vi "TopLevel.vi"() -> ()   [LabVIEW 2023]
uses:
  Test-Programs/LabVIEW Data/Common VIs/Logging/TDMSFileProperties.ctl
  <vilib>/drjdpowell/Messenging/Core Messengers/EventMessenger/EventMessenger.lvclass
  C:/Program Files (x86)/National Instruments/LabVIEW 2023/vi.lib/drjdpowell/Messenging/Core Messengers/Send/Send.lvclass
  <vilib>/drjdpowell/Messenging/Useful Actors/Metronome/Metronome.lvclass
  <vilib>/Utility/config.llb/Config Data RefNum.ctl
  <vilib>/drjdpowell/Messenging/Parallel Process/Actor type 2/Actor type2.lvclass
  <vilib>/drjdpowell/Messenging/Core Messages/Message/MSG.lvclass
  Test-Programs/LabVIEW Data/Common VIs/LoggingActor/DataLogger/DataLogger.lvclass
  C:/Program Files (x86)/National Instruments/LabVIEW 2023/vi.lib/drjdpowell/Messenging/Parallel Process/Actor type 2/Actor type2.lvclass
  Test-Programs/LabVIEW Data/HardwareActors/LabJack/LabJack.lvclass
  <vilib>/drjdpowell/Messenging/Observer/Message Translation/LabelPrefix Folder/LabelPrefix.lvclass/LabelPrefix.ctl
  <vilib>/drjdpowell/Messenging/Observer/ObserverSet/ObserverSet.lvclass/ObserverSet.ctl
  <vilib>/drjdpowell/Messenging/Observer/Observer (Parent)/Observer.lvclass/Observer.ctl
  <vilib>/drjdpowell/Messenging/Core Messages/Message/MSG.lvclass/MSG.ctl
  <vilib>/drjdpowell/Messenging/Core Messages/VarMessage/VariantMSG.lvclass/VariantMSG.ctl
  <vilib>/drjdpowell/Messenging/Core Messages/ErrorMessage/ErrorMSG.lvclass/ErrorMSG.ctl
  <vilib>/drjdpowell/Messenging/ObserverRegister/ObserverRegistry.lvclass/ObserverRegistry.ctl
  232e0ddc-f0a7-475d-9058-5032f8458813.vi
  4898256e-b016-494f-9508-2ceef4e6911c.vi
  fbe48fe1-a9cb-4763-93ba-57ead91cbc6a.vi
  <vilib>/drjdpowell/Messenging/Observer/ObserverSet/Prefix Messages.vi
  da9fa938-703e-4c08-9a98-6a32d2093df5.vi
  9b4254ec-8474-4d97-9ca8-57f430c7d8e7.vi
  0a5995e6-4927-490a-bb37-60573358c305.vi
  110a24bf-4286-4484-b55a-b16bf2ec8831.vi
  1f5a9617-5d79-4e61-ab12-c2058fb64140.vi
  cfb725ca-ad06-4a59-ac7e-8d4b7f4c84e1.vi
  9016b64b-a8fb-4694-8e11-e9e188559255.vi
  86903c63-ab96-464e-805c-7ef89f07dfc2.vi
  d424b141-51df-465e-96e3-0435ae11a4e9.vi
  6f407243-e5cf-4ee0-b394-424fafddb9ed.vi
  <vilib>/drjdpowell/Messenging/Core Messages/Message/Read Message Label (faster).vi
  <vilib>/drjdpowell/Messenging/Observer/Message Translation/LabelPrefix Folder/Prefix.vi
  <vilib>/drjdpowell/Messenging/Observer/ObserverSet/Add Translator.vi
  da9fa938-703e-4c08-9a98-6a32d2093df5.vi/afc9f7b6-782e-46b2-95da-8e576e84c933.vi
  9b4254ec-8474-4d97-9ca8-57f430c7d8e7.vi/afc9f7b6-782e-46b2-95da-8e576e84c933.vi
  0a5995e6-4927-490a-bb37-60573358c305.vi/afc9f7b6-782e-46b2-95da-8e576e84c933.vi
  110a24bf-4286-4484-b55a-b16bf2ec8831.vi/afc9f7b6-782e-46b2-95da-8e576e84c933.vi
  1f5a9617-5d79-4e61-ab12-c2058fb64140.vi/afc9f7b6-782e-46b2-95da-8e576e84c933.vi
  cfb725ca-ad06-4a59-ac7e-8d4b7f4c84e1.vi/afc9f7b6-782e-46b2-95da-8e576e84c933.vi
  9016b64b-a8fb-4694-8e11-e9e188559255.vi/afc9f7b6-782e-46b2-95da-8e576e84c933.vi
  86903c63-ab96-464e-805c-7ef89f07dfc2.vi/afc9f7b6-782e-46b2-95da-8e576e84c933.vi
  d424b141-51df-465e-96e3-0435ae11a4e9.vi/afc9f7b6-782e-46b2-95da-8e576e84c933.vi
  6f407243-e5cf-4ee0-b394-424fafddb9ed.vi/afc9f7b6-782e-46b2-95da-8e576e84c933.vi
  <vilib>/drjdpowell/Messenging/Core Messages/Message/Get Label (internal).vi
  <vilib>/drjdpowell/Messenging/Observer/ObserverSet/Write Array of Observers.vi
  <vilib>/drjdpowell/Messenging/Observer/Observer (Parent)/Make Observer.vi
  <vilib>/drjdpowell/Messenging/Core Messages/VarMessage/Write VariantMSG.vi
  <vilib>/drjdpowell/Messenging/Core Messages/Message/Overwrite Reply Address.vi
  <vilib>/drjdpowell/Messenging/Core Messages/Message/Write (no data).vi
  <vilib>/drjdpowell/Messenging/Core Messages/ErrorMessage/Write ErrorMessage.vi
  <vilib>/drjdpowell/Messenging/Core Messages/Message/Label Message.vi
  <vilib>/drjdpowell/Messenging/Observer/Message Translation/LabelPrefix Folder/LabelPrefix.lvclass
  C:/Program Files (x86)/National Instruments/LabVIEW 2023/vi.lib/drjdpowell/Messenging/Observer/Message Translation/Translator/Translator.lvclass
  <vilib>/drjdpowell/Messenging/Observer/ObserverSet/ObserverSet.lvclass
  C:/Program Files (x86)/National Instruments/LabVIEW 2023/vi.lib/drjdpowell/Messenging/Observer/Observer (Parent)/Observer.lvclass
  <vilib>/drjdpowell/Messenging/Observer/Observer (Parent)/Observer.lvclass
  <vilib>/drjdpowell/Messenging/Core Messages/VarMessage/VariantMSG.lvclass
  C:/Program Files (x86)/National Instruments/LabVIEW 2023/vi.lib/drjdpowell/Messenging/Core Messages/Message/MSG.lvclass
  <vilib>/drjdpowell/Messenging/Core Messages/ErrorMessage/ErrorMSG.lvclass
  <vilib>/Utility/config.llb/Read Key (String).vi
  <vilib>/drjdpowell/Messenging/ObserverRegister/Send RegisterForAll.vi
  <vilib>/drjdpowell/Messenging/Observer/Message Translation/Translator/Translator.lvclass
  <vilib>/drjdpowell/Messenging/Core Messengers/Send/Send.lvclass
  <vilib>/drjdpowell/Messenging/ObserverRegister/Commands/ParentCommand/ObserverRegistryCommand.lvclass
  <vilib>/drjdpowell/Messenging/ObserverRegister/ObsReg.lvlib
  <vilib>/drjdpowell/Messenging/Actor Templates Support/Actor Template Support.lvlib
  <vilib>/drjdpowell/Messenging/ObserverRegister/ObserverRegistry.lvclass
  <vilib>/drjdpowell/Messenging/Core Messages/MSG Library/SendMSG.lvlib
  <vilib>/drjdpowell/Messenging/Dialog Boxes/Display Message to User/Async Display Message to User.lvclass
  <vilib>/Utility/config.llb/NI_LVConfig.lvlib
  C:/Program Files (x86)/National Instruments/LabVIEW 2023/vi.lib/drjdpowell/Messenging/Core Messengers/Messenger (Parent)/Messenger.lvclass
  C:/Program Files (x86)/National Instruments/LabVIEW 2023/vi.lib/drjdpowell/Messenging/Core Messengers/EventMessenger/EventMessenger.lvclass
  <vilib>/drjdpowell/Messenging/Observer/Observer (Parent)/Observer.lvlib
  C:/Program Files (x86)/National Instruments/LabVIEW 2023/vi.lib/drjdpowell/Messenging/Parallel Process/Actor/Actor.lvclass
panel:
  in  "Clear Graphs":bool
  in  "Tab Control":enum32{"LabJack"}(tab)
  in  "Pressure Regulator":dbl(slide) caption="PSI" scale=0.0..450.0
  in  "Connect LabJack":bool
  in  "Load":bool
  in  "Default All Current Values":bool
  in  "Reset Elapsed Time":bool
  out "Elapsed Time":dbl format="%<%H:%M:%S>t"
  out "Test In Progress":bool
  in  "End Test":bool
  in  "Start Test":bool
  in  "Test Properties":T1
  in  "Stop":bool
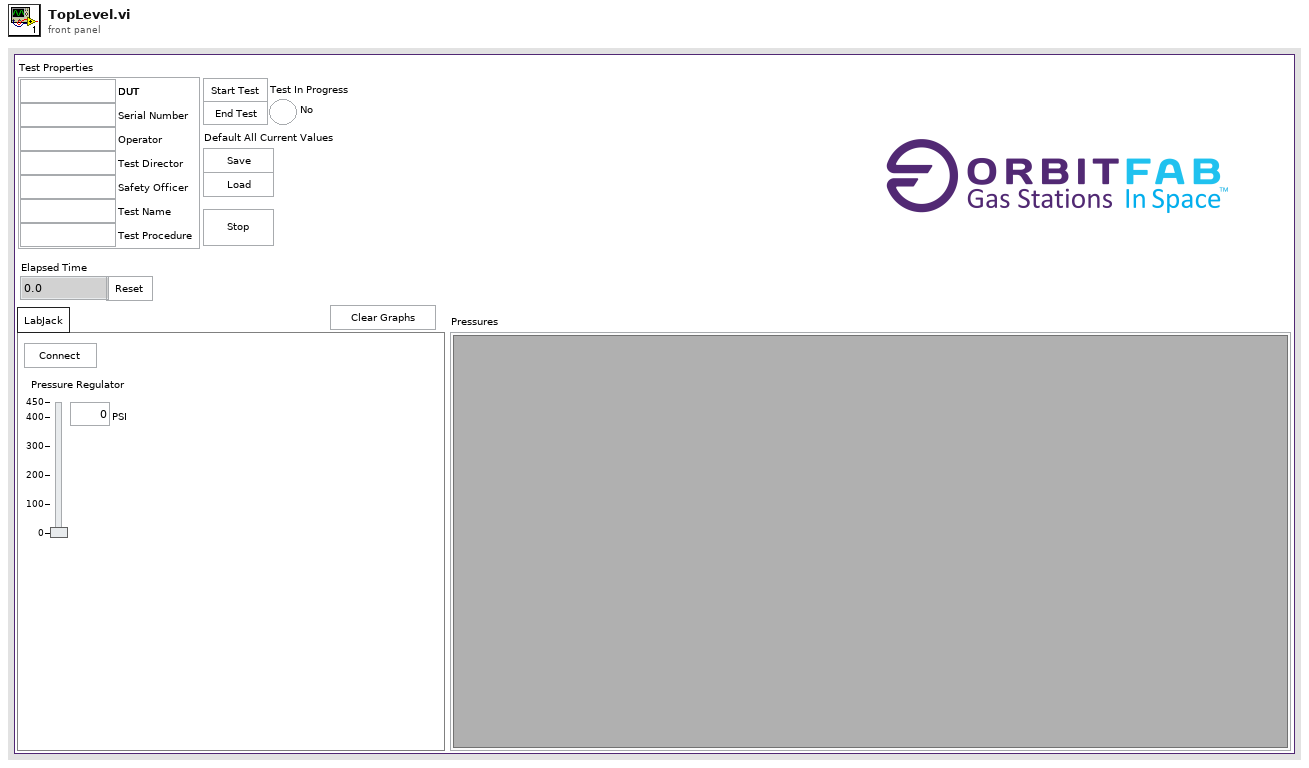
[diagram p1: front panel]
types:
  T1 = typedef "TDMSFileProperties.ctl" = cluster{"DUT":string, "Serial Number":string, "Operator":string, "Test Director":string, "Safety Officer":string, "Test Station":string, "Test Name":string, "Test Procedure":string}
  T2 = typedef "NI_LVConfig.lvlib/Config Data RefNum.ctl" = refnum<k1>
  T3 = cluster{"TopLevelMessenger":refnum<class "EventMessenger.lvclass">, "Test Status":cluster{"Test Metronome":refnum<class "Metronome.lvclass">, "Test Status":string, "Step Time":timestamp}, "App Control":cluster{"Front Panel Config refnum":T2, "This VI":refnum<vi>, "FP Metronome":refnum<class "Metronome.lvclass">, "WFM Data":waveform(dbl)[], "PT Data":dbl[]}, "DataLogger":cluster{"Actor":refnum<class "Actor type2.lvclass">, "Record Data":bool, "Data Packet":cluster{"Group Name":string, "Channel Names":string[], "Data":dbl[]}}, "EmailNotifier":cluster{"Actor":refnum<class "Actor type2.lvclass">, "Send":bool, "Last Sent":timestamp}, "LabJack":cluster{"Actor":refnum<class "Actor type2.lvclass">, "Metronome":refnum<class "Metronome.lvclass">, "Handle":u32, "Connected":bool, "t0":timestamp, "dt":dbl, "PT Data":dbl[][], "Target PSI":dbl, "PT Names":string[], "TDAC#":string}}
  T4 = cluster{"\"Message Received\" Event Reg":refnum<event-registration>}
  T5 = cluster{"Multipliers":dbl[], "Offsets":dbl[], "Names":string[]}
  T6 = cluster{"PT +Channels":string[], "PT -Channels":i32[], "PT Multipliers":dbl[], "PT Offsets":dbl[]}
  T7 = cluster{"Group Name":string, "Channel Names":string[], "Data":dbl[]}
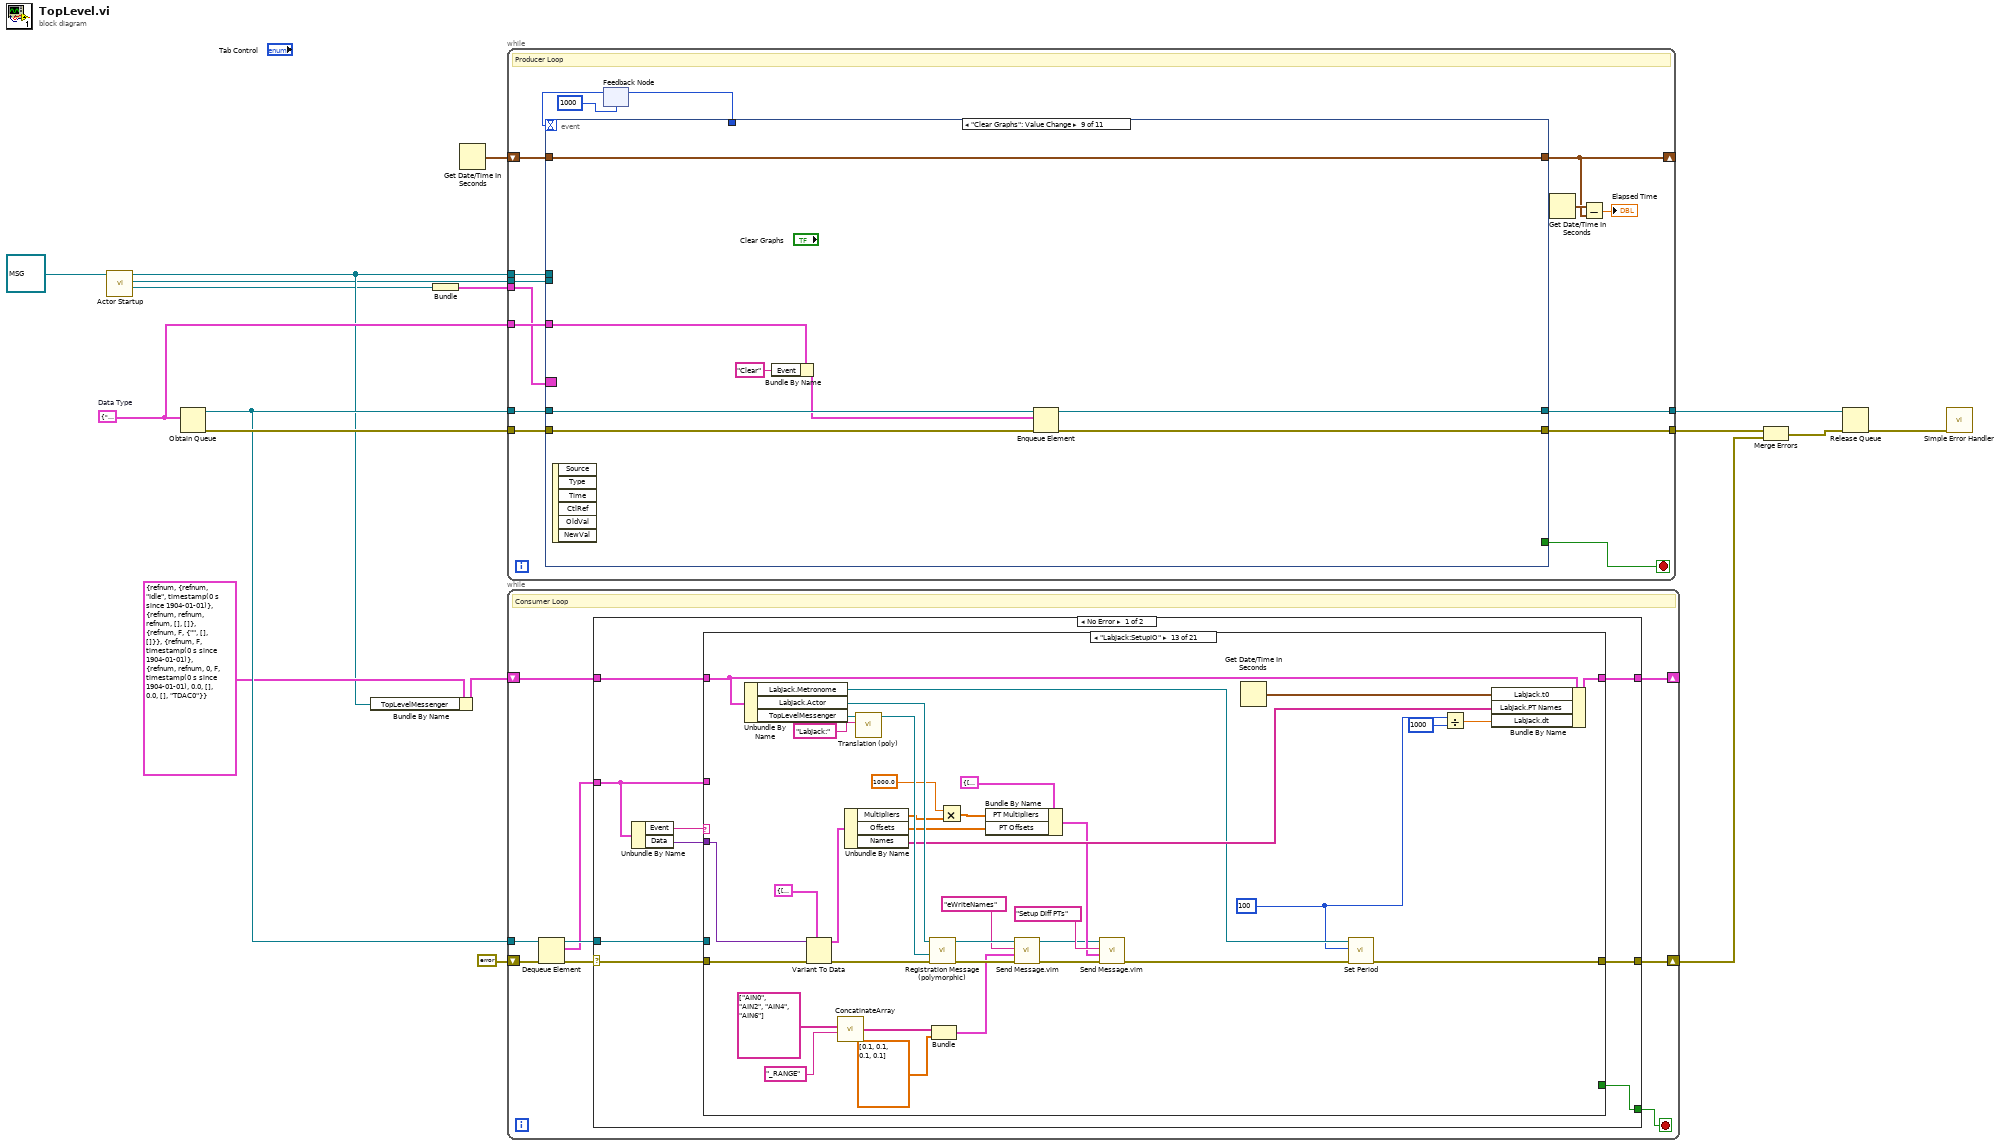
[diagram p0: block diagram]
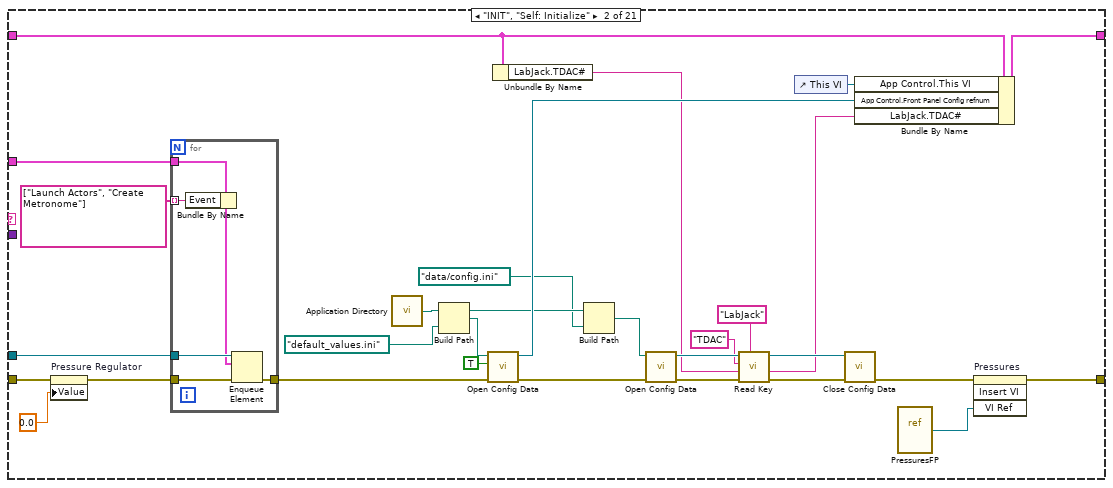
[diagram p3: hidden frame]
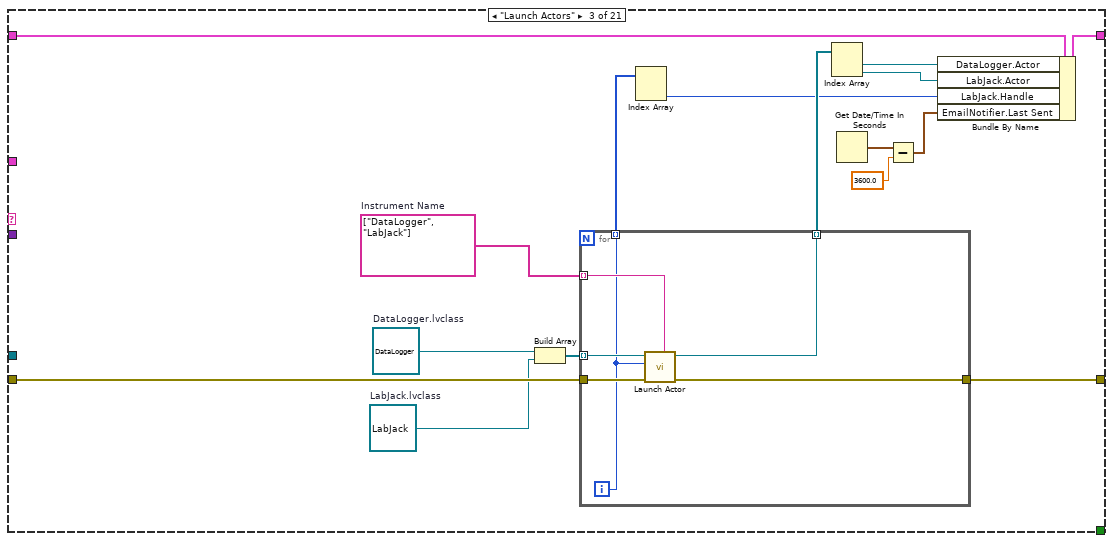
[diagram p4: hidden frame]
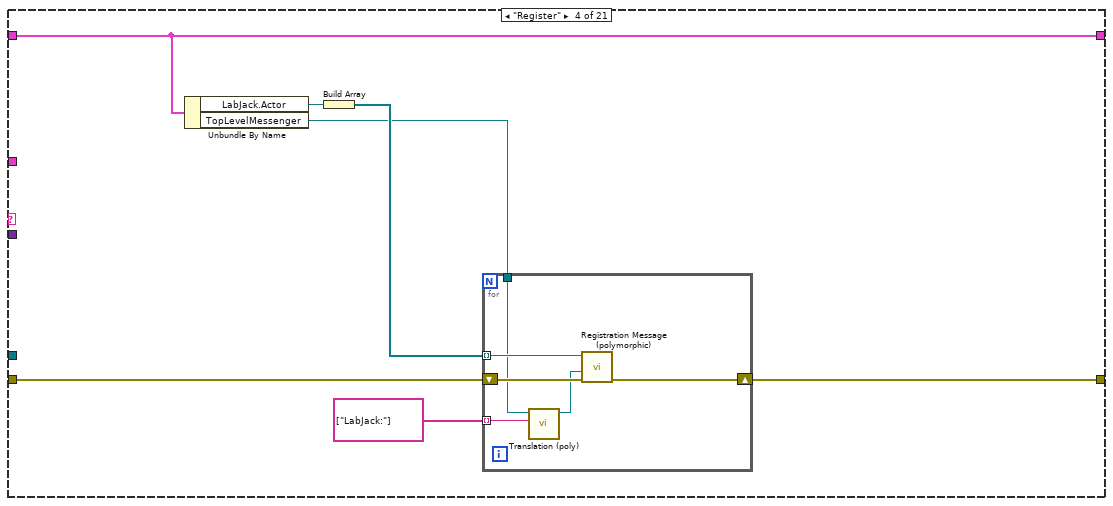
[diagram p5: hidden frame]
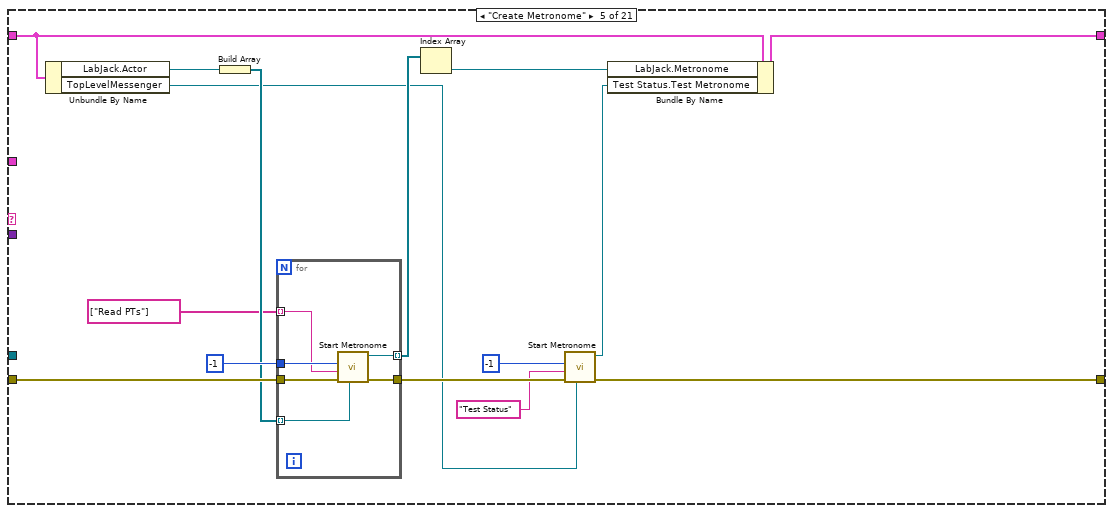
[diagram p6: hidden frame]
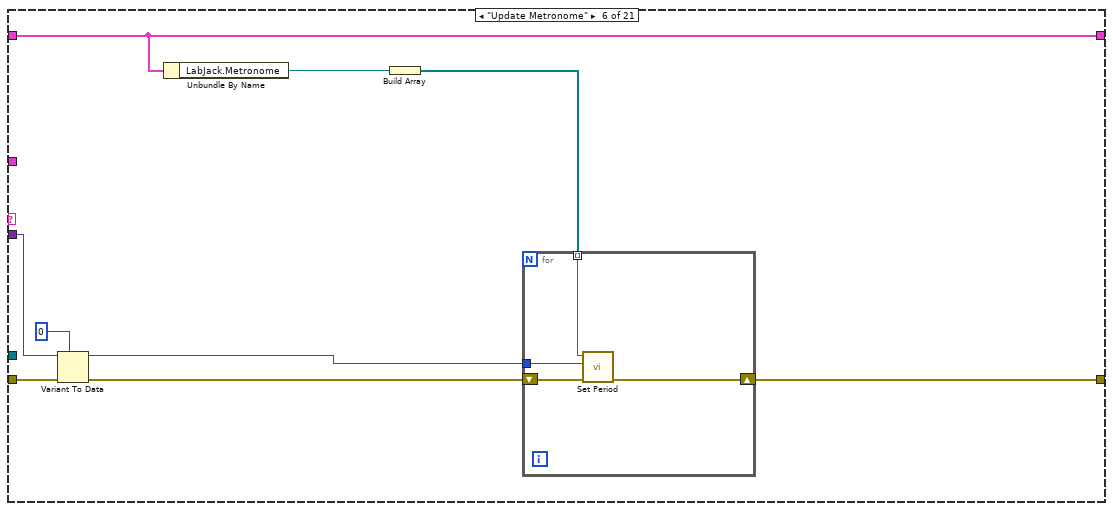
[diagram p7: hidden frame]
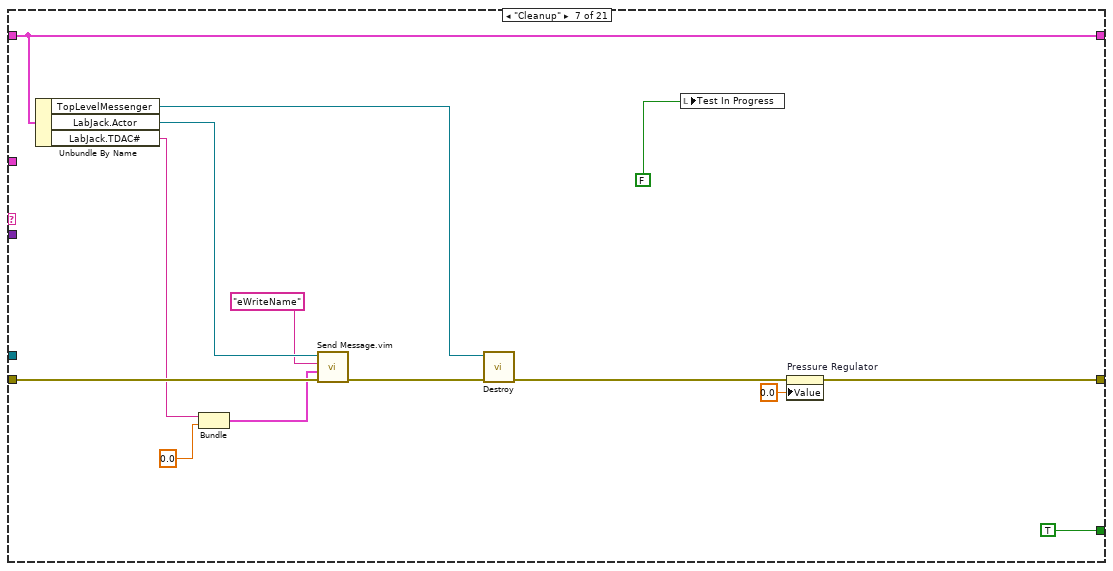
[diagram p8: hidden frame]
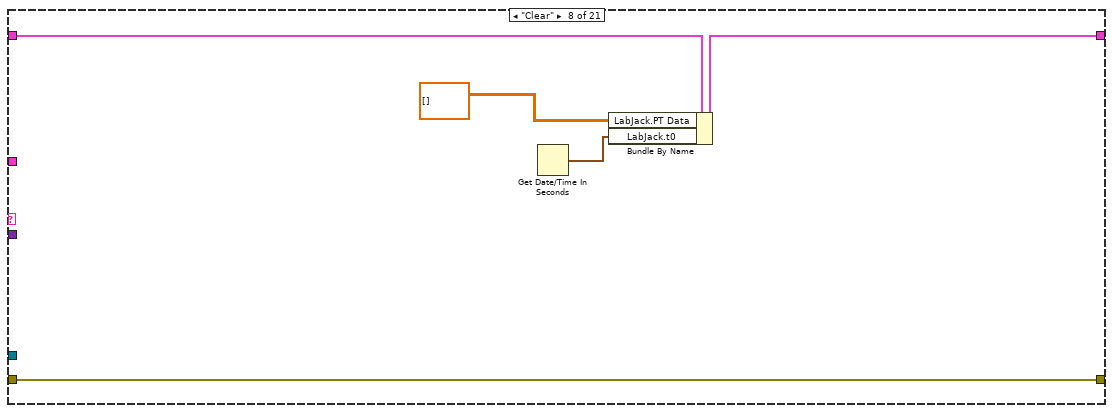
[diagram p9: hidden frame]
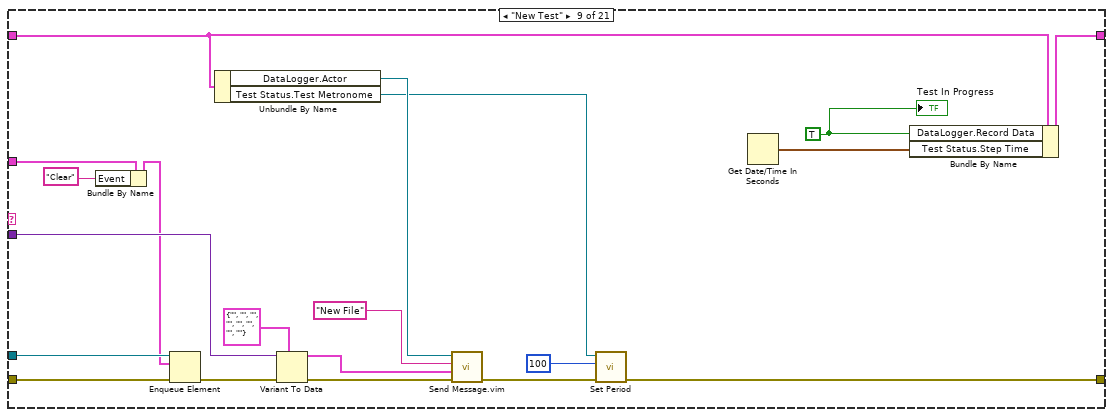
[diagram p10: hidden frame]
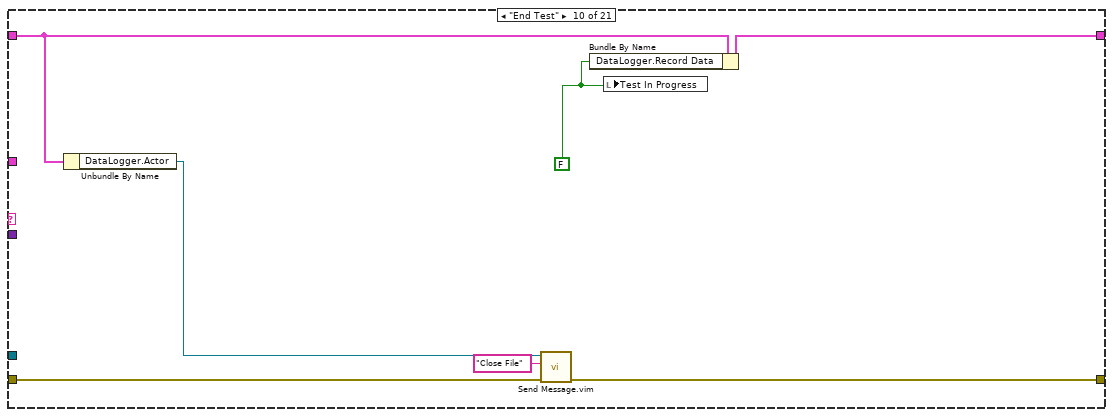
[diagram p11: hidden frame]
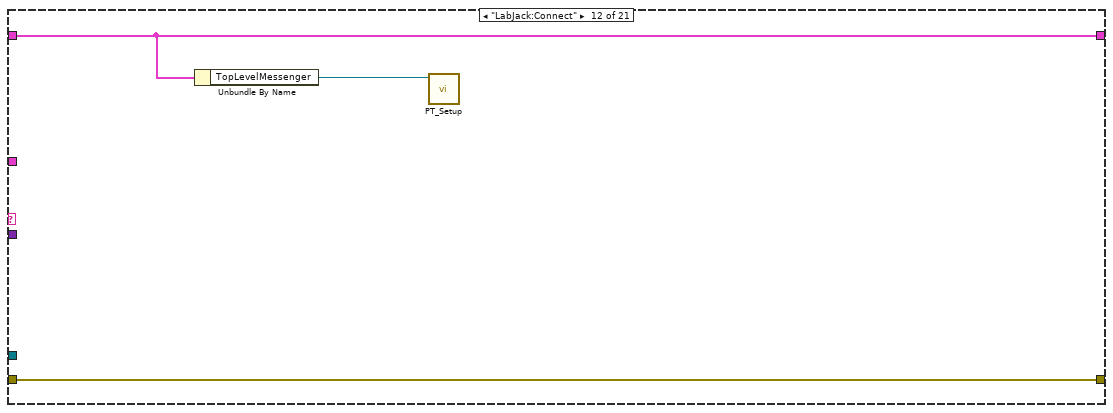
[diagram p13: hidden frame]
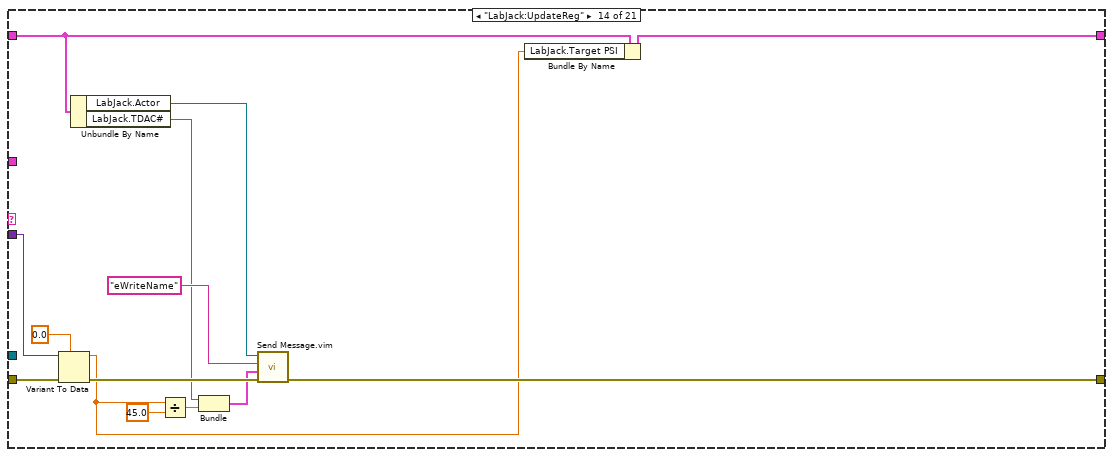
[diagram p14: hidden frame]
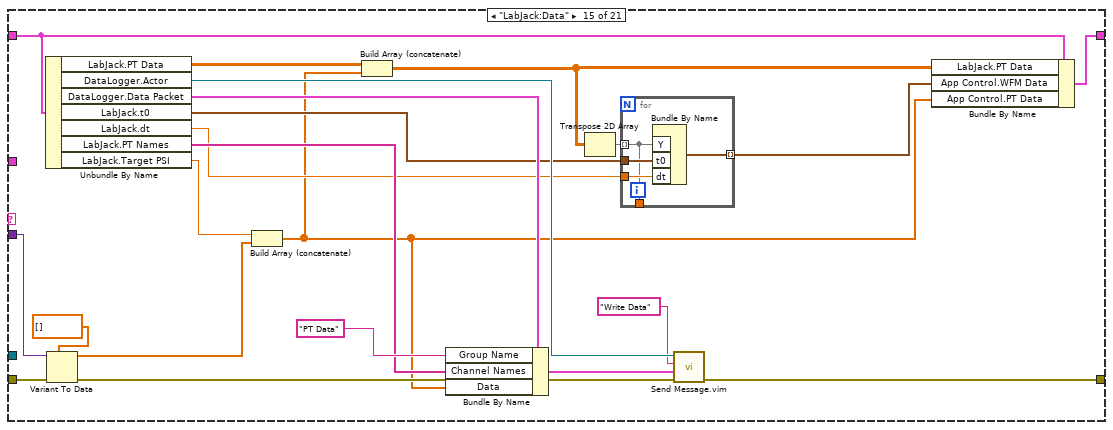
[diagram p15: hidden frame]
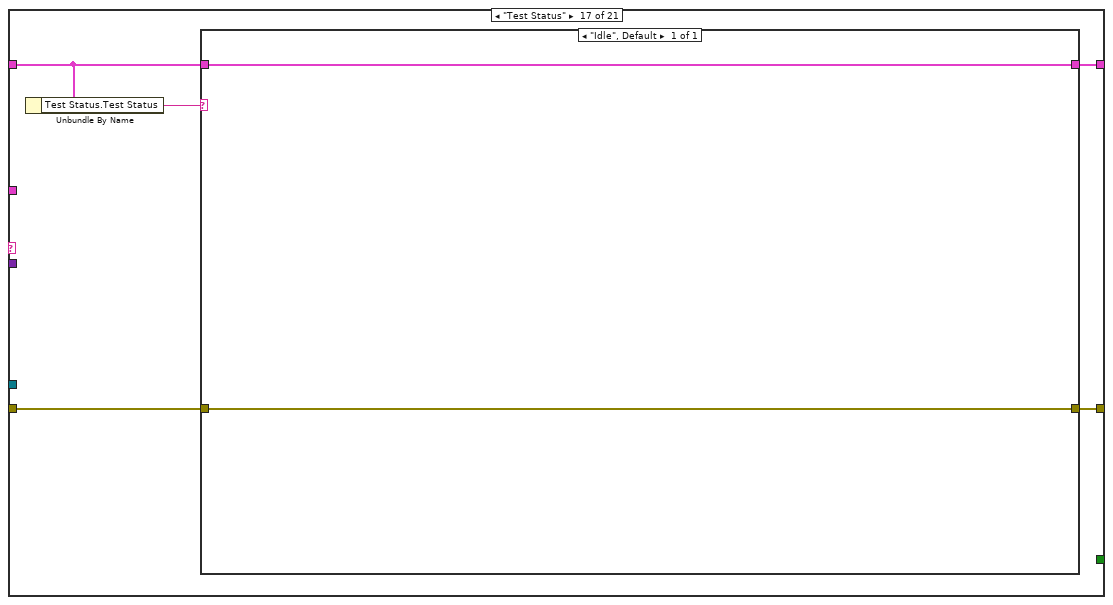
[diagram p17: hidden frame]
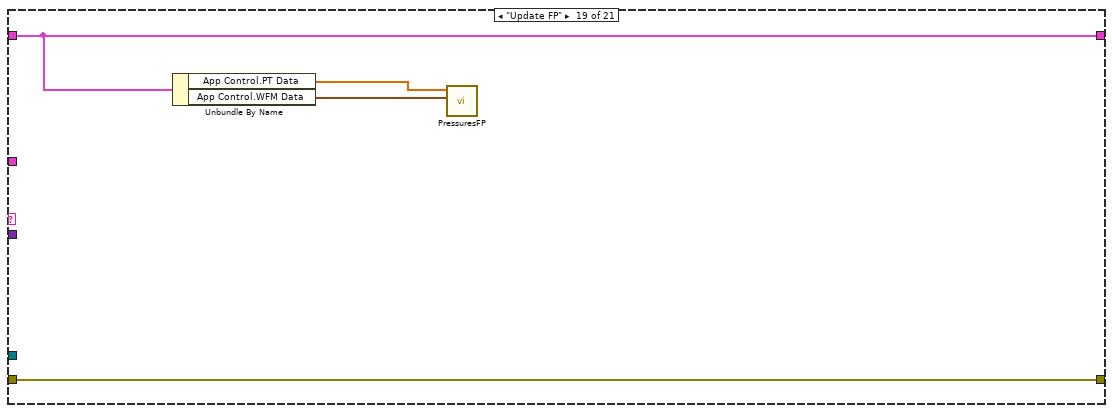
[diagram p19: hidden frame]
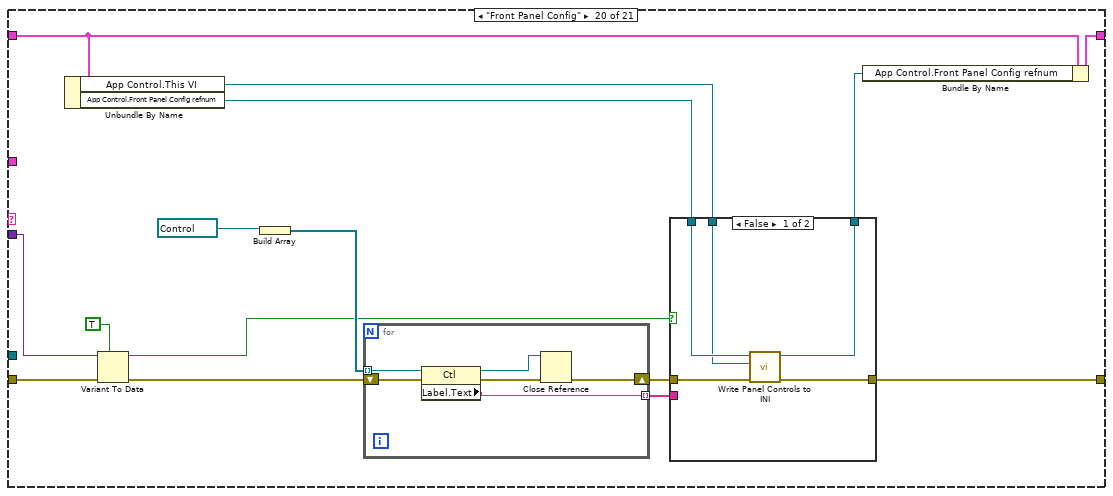
[diagram p20: hidden frame]
diagram:
  w15 = cluster{"Event":string, "Data":variant} {"Event"="", "Data"=variant}  # Data Type
  n1 = call <vilib>:"Actor Startup.vi"("Startup Message in"=refnum<class "MSG.lvclass"> refnum ("Startup Message")) -> ("\"Message Received\" Event Reg"=w3:refnum<event-registration>, "ObserverRegistry"=w4:refnum<class "ObserverRegistry.lvclass">, "Actor's Event Messenger"=w5:refnum<class "EventMessenger.lvclass">)  [unwired: 6 in, 2 out]
  n2 = Obtain Queue(element data type=w15) -> (queue out=w16:refnum<queue>, error out=w17:errorcluster)  [unwired: 4 in, 1 out]
  n3 = Bundle By Name(cluster=T3 {"TopLevelMessenger"=refnum, "Test Status"={"Test Metronome"=refnum, "Test Status"="Idle", "Step Time"=timestamp(0 s since 1904-01-01)}, "App Control"={"Front Panel Config refnum"=refnum, "This VI"=refnum, "FP Metronome"=refnum, "WFM Data"=[], "PT Data"=[]}, "DataLogger"={"Actor"=refnum, "Record Data"=FALSE, "Data Packet"={"Group Name"="", "Channel Names"=[], "Data"=[]}}, "EmailNotifier"={"Actor"=refnum, "Send"=FALSE, "Last Sent"=timestamp(0 s since 1904-01-01)}, "LabJack"={"Actor"=refnum, "Metronome"=refnum, "Handle"=0, "Connected"=FALSE, "t0"=timestamp(0 s since 1904-01-01), "dt"=0.0, "PT Data"=[], "Target PSI"=0.0, "PT Names"=[], "TDAC#"="TDAC0"}} ("Properties"), "TopLevelMessenger"=w5) -> (w8:T3)
  n4 = Bundle("\"Message Received\" Event Reg"=w3) -> (w2:T4)  [unwired: 1 in]
  n5 = Get Date/Time In Seconds() -> (seconds since 1Jan1904=w1:timestamp)
  n6 = while {
    tunnel: w16 -> [w32]
    tunnel: w15 -> [w33]
    tunnel: [w29] -> w11
    tunnel: w5 -> [w27]
    tunnel: w4 -> [w26]
    tunnel: w2 -> [w25]
    shift-right: [w21] -> _
    shift-left: w1 -> [w24]
    tunnel: w17 -> [w31]
    tunnel: [w30] -> w13
    stop <- w28 stop-if-true
    # "Producer Loop"
    n7 = feedback #1(1000) -> (w18:i32)
    n8 = event shown="[8] \"Clear Graphs\": Value Change" {
      selector: w25 -> [_ _ _ _ _ _ _ _ _ _ _]
      dyn-events: _ -> [_ _ _ _ _ _ _ _ _ _ _]
      timeout: w18 -> [_ _ _ w60 w70 w80 w90 w100 _ w168 w172]
      tunnel: w33 -> [w37 w45 w54 w64 w75 w85 w94 w102 w163 _ w176]
      tunnel: w32 -> [w39 w47 w56 w66 w76 w87 w96 w107 w164 w169 w179]
      tunnel: w31 -> [w42 w50 w59 w69 w79 w89 w98 w114 w167 w171 w183]
      tunnel: [w40 w48 w57 w67 w77 w88 w97 w108 w165 w171 w180] -> w30
      tunnel: [w38 w46 w55 w65 w72 w86 w95 w106 w162 w169 w178] -> w29
      tunnel: [_ _ _ w68 w78 _ _ w103 _ _ _] -> w28
      tunnel: w27 -> [_ _ _ _ _ _ _ _ _ _ _]
      tunnel: w26 -> [_ _ _ _ _ _ _ w112 _ _ _]
      tunnel: w24 -> [w41 w49 w58 w61 w71 w81 w91 w101 w166 _ w182]
      tunnel: [w41 w49 w58 w61 w71 w81 w91 w101 w166 w170 w182] -> w21
      tunnel: [1000 _ _ w60 w70 w80 w90 w99 _ w168 w172] -> w20
      event Timeout {
        n9 = event-data() -> ()  [unwired: 1 in, 3 out]
        n10 = Bundle By Name(cluster=w37, "Event"="Update FP") -> (w36:cluster{"Event":string, "Data":variant})
        n11 = Enqueue Element(queue=w39, element=w36, error in (no error)=w42) -> (queue out=w38:refnum<queue>, error out=w40:errorcluster)  [unwired: 1 in, 1 out]
      }
      event "Connect LabJack": Value Change {
        n12 = event-data() -> ()  [unwired: 1 in, 6 out]
        n13 = Bundle By Name(cluster=w45, "Event"="LabJack:Connect") -> (w44:cluster{"Event":string, "Data":variant})
        n14 = Enqueue Element(queue=w47, element=w44, error in (no error)=w50) -> (queue out=w46:refnum<queue>, error out=w48:errorcluster)  [unwired: 1 in, 1 out]
      }
      event "Pressure Regulator": Value Change {
        n15 = event-data() -> ("NewVal"=w51:dbl)  [unwired: 1 in, 5 out]
        n16 = Bundle By Name(cluster=w54, "Event"="LabJack:UpdateReg", "Data"=w51) -> (w53:cluster{"Event":string, "Data":variant})
        n17 = Enqueue Element(queue=w56, element=w53, error in (no error)=w59) -> (queue out=w55:refnum<queue>, error out=w57:errorcluster)  [unwired: 1 in, 1 out]
      }
      event "Stop": Value Change {
        n18 = event-data() -> ("NewVal"=w68:bool)  [unwired: 1 in, 5 out]
        n19 = Bundle By Name(cluster=w64, "Event"="Cleanup") -> (w63:cluster{"Event":string, "Data":variant})
        n20 = Enqueue Element(queue=w66, element=w63, error in (no error)=w69) -> (queue out=w65:refnum<queue>, error out=w67:errorcluster)  [unwired: 1 in, 1 out]
      }
      event Panel Close? {
        w78 = TRUE ("Discard?")
        n21 = event-data() -> ()  [unwired: 1 in, 4 out]
        n22 = Bundle By Name(cluster=w75, "Event"="Cleanup") -> (w74:cluster{"Event":string, "Data":variant})
        n23 = Enqueue Element(queue=w76, element=w74, error in (no error)=w79) -> (queue out=w72:refnum<queue>, error out=w77:errorcluster)  [unwired: 1 in, 1 out]
        n24 = event-data("Discard?"=w78) -> ()  [unwired: 1 in, 1 out]
      }
      event "Start Test": Value Change {
        n25 = event-data() -> ()  [unwired: 1 in, 6 out]
        n26 = Bundle By Name(cluster=w85, "Event"="New Test", "Data"="Test Properties") -> (w84:cluster{"Event":string, "Data":variant})
        n27 = Enqueue Element(queue=w87, element=w84, error in (no error)=w89) -> (queue out=w86:refnum<queue>, error out=w88:errorcluster)  [unwired: 1 in, 1 out]
      }
      event "End Test": Value Change {
        n28 = event-data() -> ()  [unwired: 1 in, 6 out]
        n29 = Bundle By Name(cluster=w94, "Event"="End Test") -> (w93:cluster{"Event":string, "Data":variant})
        n30 = Enqueue Element(queue=w96, element=w93, error in (no error)=w98) -> (queue out=w95:refnum<queue>, error out=w97:errorcluster)  [unwired: 1 in, 1 out]
      }
      event User Event {
        n31 = event-data() -> ("Message"=w113:refnum<class "MSG.lvclass">)  [unwired: 1 in]
        n32 = call <vilib>:"Registration.vi"("error in (no error)"=w114, "Message"=w113, "Observer Registry"=w112) -> ("error out"=w111:errorcluster, "Message (Registration messages filtered out)"=w110:refnum<class "MSG.lvclass">)  [unwired: 5 in, 2 out]
        n33 = call <vilib>:"Read Message Label.vi"("error in (no error)"=w111, "Message"=w110) -> ("error out"=w109:errorcluster, "Label"=w105:string, "Message"=w104:refnum<class "MSG.lvclass">)  [unwired: 7 in]
        n34 = case shown="\"LabJack:Read PTs\"" w105 {
          selector: w105 -> [w116 _ _ _ _]
          tunnel: w109 -> [w122 w125 w137 w149 w153]
          tunnel: [w121 w125 w133 w145 w152] -> w108
          tunnel: w107 -> [w119 w124 w131 w143 w159]
          tunnel: [w120 w124 w132 w144 w159] -> w106
          tunnel: w104 -> [_ _ w134 w146 w154]
          tunnel: [_ _ _ _ TRUE ("Discard?")] -> w103
          tunnel: w102 -> [w118 _ w130 w142 _]
          tunnel: w100 -> [w115 w123 w136 _ w150]
          tunnel: [w115 w123 w136 1 w150] -> w99
          frame Default {
            n35 = Bundle By Name(cluster=w118, "Event"=w116) -> (w117:cluster{"Event":string, "Data":variant})
            n36 = Enqueue Element(queue=w119, element=w117, error in (no error)=w122) -> (queue out=w120:refnum<queue>, error out=w121:errorcluster)  [unwired: 1 in, 1 out]
          }
          frame "Self: Initialize " {
          }
          frame "PT Constants" {
            n37 = call "Extract Message Contents.vim"("error in (no error)"=w137, "DataType and Default Value"=T5 {"Multipliers"=[], "Offsets"=[], "Names"=[]}, "Message in"=w134) -> ("error out"=w135:errorcluster, "Contents"=w127:T5)  [unwired: 5 in, 2 out]
            n38 = Bundle By Name(cluster=w130, "Event"="LabJack:SetupIO", "Data"=w127) -> (w129:cluster{"Event":string, "Data":variant})
            n39 = Enqueue Element(queue=w131, element=w129, error in (no error)=w135) -> (queue out=w132:refnum<queue>, error out=w133:errorcluster)  [unwired: 1 in, 1 out]
          }
          frame "LabJack:Read PTs" {
            n40 = call "Extract Message Contents.vim"("error in (no error)"=w149, "DataType and Default Value"=dbl[] [] ("data"), "Message in"=w146) -> ("error out"=w147:errorcluster, "Contents"=w139:dbl[])  [unwired: 5 in, 2 out]
            n41 = Bundle By Name(cluster=w142, "Event"="LabJack:Data", "Data"=w139) -> (w141:cluster{"Event":string, "Data":variant})
            n42 = Enqueue Element(queue=w143, element=w141, error in (no error)=w147) -> (queue out=w144:refnum<queue>, error out=w145:errorcluster)  [unwired: 1 in, 1 out]
          }
          frame "Consumer Error" {
            n43 = call "Extract Message Contents.vim"("error in (no error)"=w153, "DataType and Default Value"=errorcluster {"status"=FALSE, "code"=0, "source"=""} ("error out"), "Message in"=w154) -> ("error out"=w158:errorcluster, "Contents"=w155:errorcluster)  [unwired: 5 in, 2 out]
            n44 = call <vilib>:"Async Display Message to User.vi"("displayed message"="Error encountered in Consumer Loop.") -> ()  [unwired: 10 in, 1 out]
            n45 = Merge Errors(w155, w158) -> (w152:errorcluster)
          }
        }
      }
      event "Clear Graphs": Value Change {
        n46 = event-data() -> ()  [unwired: 1 in, 6 out]
        n47 = Bundle By Name(cluster=w163, "Event"="Clear") -> (w161:cluster{"Event":string, "Data":variant})
        n48 = Enqueue Element(queue=w164, element=w161, error in (no error)=w167) -> (queue out=w162:refnum<queue>, error out=w165:errorcluster)  [unwired: 1 in, 1 out]
      }
      event "Reset Elapsed Time": Value Change {
        n49 = event-data() -> ()  [unwired: 1 in, 6 out]
        n50 = Get Date/Time In Seconds() -> (seconds since 1Jan1904=w170:timestamp)
      }
      event "Default All Current Values", "Load": Value Change {
        n51 = event-data() -> ("CtlRef"=w174:refnum<vi>)  [unwired: 1 in, 5 out]
        n52 = control-ref of="Load"() -> (w175:refnum<vi>)
        n53 = Equal?(x=w174, y=w175) -> (x = y?=w173:bool)
        n54 = Bundle By Name(cluster=w176, "Event"="Front Panel Config", "Data"=w173) -> (w177:cluster{"Event":string, "Data":variant})
        n55 = Enqueue Element(queue=w179, element=w177, error in (no error)=w183) -> (queue out=w178:refnum<queue>, error out=w180:errorcluster)  [unwired: 1 in, 1 out]
      }
    }
    n56 = feedback-in #1(w20) -> ()
    n57 = Get Date/Time In Seconds() -> (seconds since 1Jan1904=w22:timestamp)
    n58 = Subtract(x=w22, y=w21) -> (x-y=→"Elapsed Time":dbl)
  }
  n59 = while {
    tunnel: w16 -> [w192]
    shift-right: [w189] -> w14
    shift-left: errorcluster {"status"=FALSE, "code"=0, "source"=""} ("error IO") -> [w191]
    shift-right: [w184] -> _
    shift-left: w8 -> [w185]
    stop <- w186 stop-if-true
    # "Consumer Loop"
    n60 = Dequeue Element(queue=w192, error in (no error)=w191) -> (queue out=w188:refnum<queue>, element=w187:cluster{"Event":string, "Data":variant}, error out=w190:errorcluster)  [unwired: 1 in, 1 out]
    n61 = case shown="No Error" w190 {
      selector: w190 -> [w198 w496]
      tunnel: [w199 w493] -> w189
      tunnel: w188 -> [w197 w492]
      tunnel: w187 -> [w193 w495]
      tunnel: [w194 FALSE] -> w186
      tunnel: w185 -> [w196 w501]
      tunnel: [w195 w501] -> w184
      frame No Error {
        n62 = Unbundle By Name(w193) -> ("Event"=w201:string, "Data"=w200:variant)
        n63 = case shown="\"LabJack:SetupIO\"" w201 {
          tunnel: w200 -> [_ _ _ _ _ w301 _ _ w345 _ _ _ w383 w406 w429 _ _ _ _ w457 _]
          tunnel: [w203 w221 w254 w266 w279 w298 w309 w324 w330 w351 w355 w358 w374 w404 w425 w436 w438 w445 w449 w460 w485] -> w199
          tunnel: w198 -> [w203 w232 w253 w267 w288 w303 w321 w324 w346 w353 w355 w358 w394 w408 w430 w436 w439 w445 w449 w461 w491]
          tunnel: w197 -> [_ w231 _ _ _ _ _ _ w338 _ _ _ _ _ _ _ _ _ _ _ _]
          tunnel: w196 -> [w202 w209 w250 w265 w287 w299 w319 w326 w342 w352 w354 w357 w392 w403 w422 w435 w441 w444 w448 w459 w489]
          tunnel: [w202 w224 w249 w265 w286 w299 w319 w325 w340 w349 w354 w357 w389 w398 w426 w435 w440 w444 w448 w451 w489] -> w195
          tunnel: [_ _ _ _ _ _ TRUE _ _ _ _ _ _ _ _ _ _ _ _ _ _] -> w194
          tunnel: w193 -> [_ w228 _ _ _ _ _ _ w337 _ _ _ _ _ _ _ _ _ _ _ _]
          frame Default {
          }
          frame "INIT", "Self: Initialize" {
            n64 = property on="Pressure Regulator" class="Slide (strict)"(error in=w232, "Value"=0.0 ("Pressure Regulator")) -> (error out=w205:errorcluster)  [unwired: 1 in, 1 out]
            n65 = for {
              tunnel: w231 -> [w237]
              tunnel: string[] ["Launch Actors", "Create Metronome"] ("Event") -> [w235] mode=indexing
              tunnel: w228 -> [w233]
              tunnel: w205 -> [w238]
              tunnel: [w234] -> w229
              n66 = Bundle By Name(cluster=w233, "Event"=w235) -> (w236:cluster{"Event":string, "Data":variant})
              n67 = Enqueue Element(queue=w237, element=w236, error in (no error)=w238) -> (error out=w234:errorcluster)  [unwired: 1 in, 2 out]
            }
            n68 = call <vilib>:"Application Directory.vi"() -> ("Application Directory"=w217:path)
            n69 = Build Path(base path=w217, name or relative path=path "default_values.ini") -> (appended path=w225:path)
            n70 = call <vilib>:"Open Config Data.vi"("error in (no error)"=w229, "create file if necessary (T)"=TRUE, "configuration file path"=w225) -> ("error out"=w219:errorcluster, "refnum"=w223:T2)  [unwired: 6 in, 1 out]
            n71 = Unbundle By Name(w209) -> ("LabJack.TDAC#"=w208:string)
            n72 = Build Path(base path=w217, name or relative path=path "data/config.ini") -> (appended path=w215:path)
            n73 = call <vilib>:"Open Config Data.vi"("error in (no error)"=w219, "configuration file path"=w215) -> ("error out"=w218:errorcluster, "refnum"=w213:T2)  [unwired: 7 in, 1 out]
            n74 = call-poly <vilib>:"Read Key.vi"("section"="LabJack", "error in (no error)"=w218, "default value"=w208, "key"="TDAC", "refnum"=w213) -> ("error out"=w214:errorcluster, "value"=w210:string, "refnum out"=w211:T2)  [unwired: 3 in, 1 out]
            n75 = control-ref of="This VI"() -> (w222:refnum<vi>)
            n76 = call <vilib>:"Close Config Data.vi"("error in (no error)"=w214, "refnum"=w211) -> ("error out"=w212:errorcluster)  [unwired: 8 in, 1 out]
            n77 = Bundle By Name(cluster=w209, "App Control.This VI"=w222, "App Control.Front Panel Config refnum"=w223, "LabJack.TDAC#"=w210) -> (w224:T3)
            n78 = vi-ref "PressuresFP.vi"() -> (w220:refnum<vi>)
            n79 = invoke on="Pressures" class="SubPnl" method="Insert VI"(error in=w212, "VI Ref"=w220) -> (error out=w221:errorcluster)  [unwired: 2 in, 3 out]
          }
          frame "Launch Actors" {
            w240 = refnum<class "LabJack.lvclass"> refnum  # LabJack.lvclass
            w244 = refnum<class "DataLogger.lvclass"> refnum  # DataLogger.lvclass
            w251 = string[] ["DataLogger", "LabJack"]  # Instrument Name
            n80 = Build Array(w244, w240) -> (w252:refnum<class "Actor type2.lvclass">[])
            n81 = for {
              tunnel: w252 -> [w258] mode=indexing
              tunnel: w251 -> [w257] mode=indexing
              tunnel: [w256] -> w248 mode=indexing
              tunnel: [w255] -> w247 mode=indexing
              tunnel: w253 -> [w259]
              tunnel: [w260] -> w254
              i -> [w255]
              n82 = call-dynamic "Launch Actor.vi"("Actor Description"=w257, "error in (no error)"=w259, "Startup Parameters"=w255, "Actor Type"=w258) -> ("error out"=w260:errorcluster, "Running Actor out"=w256:refnum<class "Actor type2.lvclass">)  [unwired: 6 in]
            }
            n83 = Index Array(array=w247) -> (element #2=w245:i32)  [unwired: 2 in, 1 out]
            n84 = Index Array(array=w248) -> (element #1=w246:refnum<class "Actor type2.lvclass">, element #2=w239:refnum<class "Actor type2.lvclass">)  [unwired: 2 in]
            n85 = Get Date/Time In Seconds() -> (seconds since 1Jan1904=w243:timestamp)
            n86 = Subtract(x=w243, y=3600.0) -> (x-y=w242:timestamp)
            n87 = Bundle By Name(cluster=w250, "DataLogger.Actor"=w246, "LabJack.Actor"=w239, "LabJack.Handle"=w245, "EmailNotifier.Last Sent"=w242) -> (w249:T3)
          }
          frame "Register" {
            n88 = Unbundle By Name(w265) -> ("LabJack.Actor"=w264:refnum<class "Actor type2.lvclass">, "TopLevelMessenger"=w262:refnum<class "EventMessenger.lvclass">)
            n89 = Build Array(w264) -> (w263:refnum<class "Actor type2.lvclass">[])
            n90 = for {
              tunnel: w263 -> [w272] mode=indexing
              shift-right: [w273] -> w266
              shift-left: w267 -> [w271]
              tunnel: w262 -> [w270]
              tunnel: string[] ["LabJack:"] ("Prefix message labels with") -> [w268] mode=indexing
              n91 = call-poly <vilib>:"Translation (poly).vi"("Prefix message labels with"=w268, "Address"=w270) -> ("Observer Address"=w269:refnum<class "Observer.lvclass">)  [unwired: 9 in]
              n92 = call-poly <vilib>:"Registration Message (polymorphic).vi"("error in (no error)"=w271, "Address to Register"=w269, "Address to Register With"=w272) -> ("error out"=w273:errorcluster)  [unwired: 7 in, 1 out]
            }
          }
          frame "Create Metronome" {
            n93 = Unbundle By Name(w287) -> ("LabJack.Actor"=w284:refnum<class "Actor type2.lvclass">, "TopLevelMessenger"=w276:refnum<class "EventMessenger.lvclass">)
            n94 = Build Array(w284) -> (w283:refnum<class "Actor type2.lvclass">[])
            n95 = for {
              tunnel: w288 -> [w294]
              tunnel: -1 ("Initial Period (ms)") -> [w293]
              tunnel: w283 -> [w290] mode=indexing
              tunnel: [w292] -> w281 mode=indexing
              tunnel: [w291] -> w282
              tunnel: string[] ["Read PTs"] ("Relabel \"MetronomeTick\" messages") -> [w289] mode=indexing
              n96 = call <vilib>:"Start Metronome.vi"("Address for \"MetronomeTick\" messages"=w290, "error in (no error)"=w294, "Relabel \"MetronomeTick\" messages"=w289, "Initial Period (ms)"=w293) -> ("error out"=w291:errorcluster, "Metronome out"=w292:refnum<class "Metronome.lvclass">)  [unwired: 6 in]
            }
            n97 = Index Array(array=w281) -> (element=w280:refnum<class "Metronome.lvclass">)  [unwired: 1 in]
            n98 = call <vilib>:"Start Metronome.vi"("Address for \"MetronomeTick\" messages"=w276, "error in (no error)"=w282, "Relabel \"MetronomeTick\" messages"="Test Status" ("Relabel \"MetronomeTick\" messages"), "Initial Period (ms)"=-1) -> ("error out"=w279:errorcluster, "Metronome out"=w275:refnum<class "Metronome.lvclass">)  [unwired: 6 in]
            n99 = Bundle By Name(cluster=w287, "LabJack.Metronome"=w280, "Test Status.Test Metronome"=w275) -> (w286:T3)
          }
          frame "Update Metronome" {
            n100 = Variant To Data(error in=w303, type=u32 0 ("Samples per second"), Variant=w301) -> (data=w296:u32, error out=w302:errorcluster)
            n101 = Unbundle By Name(w299) -> ("LabJack.Metronome"=w297:refnum<class "Metronome.lvclass">)
            n102 = Build Array(w297) -> (w295:refnum<class "Metronome.lvclass">[])
            n103 = for {
              tunnel: w295 -> [w305] mode=indexing
              shift-right: [w306] -> w298
              shift-left: w302 -> [w307]
              tunnel: w296 -> [w304]
              n104 = call <vilib>:"Set Period.vi"("error in (no error)"=w307, "Period (ms)"=w304, "Metronome in"=w305) -> ("error out"=w306:errorcluster)  [unwired: 7 in, 1 out]
            }
          }
          frame "Cleanup" {
            n105 = Unbundle By Name(w319) -> ("TopLevelMessenger"=w318:refnum<class "EventMessenger.lvclass">, "LabJack.Actor"=w314:refnum<class "Actor type2.lvclass">, "LabJack.TDAC#"=w312:string)
            n106 = Bundle("TDAC#"=w312, 0.0) -> (w310:cluster{"TDAC#":string, dbl})  [unwired: 1 in]
            n107 = call "Send Message.vim"("error in (no error)"=w321, "Contents"=w310, "Label or Message"="eWriteName", "Address"=w314) -> ("error out"=w315:errorcluster)  [unwired: 6 in, 1 out]
            n108 = call-dynamic "Destroy.vi"("error in (no error)"=w315, "EventMessenger in"=w318) -> ("error out"=w316:errorcluster)  [unwired: 9 in]
            n109 = local write "Test In Progress"(FALSE ("Connect PSU")) -> ()
            n110 = property on="Pressure Regulator" class="Slide (strict)"(error in=w316, "Value"=0.0 ("Pressure Regulator")) -> (error out=w309:errorcluster)  [unwired: 1 in, 1 out]
          }
          frame "Clear" {
            n111 = Get Date/Time In Seconds() -> (seconds since 1Jan1904=w322:timestamp)
            n112 = Bundle By Name(cluster=w326, "LabJack.PT Data"=dbl[][] [] ("DAQ 1"), "LabJack.t0"=w322) -> (w325:T3)
          }
          frame "New Test" {
            w341 = TRUE ("Record Data")
            n113 = Bundle By Name(cluster=w337, "Event"="Clear") -> (w336:cluster{"Event":string, "Data":variant})
            n114 = Enqueue Element(queue=w338, element=w336, error in (no error)=w346) -> (error out=w339:errorcluster)  [unwired: 1 in, 2 out]
            n115 = Unbundle By Name(w342) -> ("DataLogger.Actor"=w332:refnum<class "Actor type2.lvclass">, "Test Status.Test Metronome"=w329:refnum<class "Metronome.lvclass">)
            n116 = Variant To Data(error in=w339, type=T1 {"DUT"="", "Serial Number"="", "Operator"="", "Test Director"="", "Safety Officer"="", "Test Station"="", "Test Name"="", "Test Procedure"=""} ("Test Properties"), Variant=w345) -> (data=w333:T1, error out=w343:errorcluster)
            n117 = call "Send Message.vim"("error in (no error)"=w343, "Contents"=w333, "Label or Message"="New File", "Address"=w332) -> ("error out"=w334:errorcluster)  [unwired: 6 in, 1 out]
            n118 = call <vilib>:"Set Period.vi"("error in (no error)"=w334, "Period (ms)"=100, "Metronome in"=w329) -> ("error out"=w330:errorcluster)  [unwired: 7 in, 1 out]
            n119 = Get Date/Time In Seconds() -> (seconds since 1Jan1904=w327:timestamp)
            n120 = Bundle By Name(cluster=w342, "DataLogger.Record Data"=w341, "Test Status.Step Time"=w327) -> (w340:T3)
            "Test In Progress" <- w341
          }
          frame "End Test" {
            w348 = FALSE ("Record Data")
            n121 = Unbundle By Name(w352) -> ("DataLogger.Actor"=w350:refnum<class "Actor type2.lvclass">)
            n122 = call "Send Message.vim"("error in (no error)"=w353, "Label or Message"="Close File", "Address"=w350) -> ("error out"=w351:errorcluster)  [unwired: 7 in, 1 out]
            n123 = Bundle By Name(cluster=w352, "DataLogger.Record Data"=w348) -> (w349:T3)
            n124 = local write "Test In Progress"(w348) -> ()
          }
          frame "----------LabJack Actions----------" {
          }
          frame "LabJack:Connect" {
            n125 = Unbundle By Name(w357) -> ("TopLevelMessenger"=w356:refnum<class "EventMessenger.lvclass">)
            n126 = call "PT_Setup.vi"("Actor's Event Messenger"=w356) -> ()  [unwired: 11 in]
          }
          frame "LabJack:SetupIO" {
            w372 = 100 ("Period (ms)")
            n127 = Unbundle By Name(w392) -> ("LabJack.Metronome"=w373:refnum<class "Metronome.lvclass">, "LabJack.Actor"=w391:refnum<class "Actor type2.lvclass">, "TopLevelMessenger"=w390:refnum<class "EventMessenger.lvclass">)
            n128 = Variant To Data(error in=w394, type=T5 {"Multipliers"=[], "Offsets"=[], "Names"=[]}, Variant=w383) -> (data=w380:T5, error out=w384:errorcluster)
            n129 = call "ConcatinateArray.vi"("Input Array"=string[] ["AIN0", "AIN2", "AIN4", "AIN6"], "Concatenated String"="_RANGE") -> ("Output Array"=w363:string[])  [unwired: 3 in]
            n130 = Unbundle By Name(w380) -> ("Multipliers"=w377:dbl[], "Offsets"=w376:dbl[], "Names"=w379:string[])
            n131 = call-poly <vilib>:"Translation (poly).vi"("Prefix message labels with"="LabJack:", "Address"=w390) -> ("Observer Address"=w387:refnum<class "Observer.lvclass">)  [unwired: 9 in]
            n132 = call-poly <vilib>:"Registration Message (polymorphic).vi"("error in (no error)"=w384, "Address to Register"=w387, "Address to Register With"=w391) -> ("error out"=w393:errorcluster, "Address"=w368:refnum<class "Actor type2.lvclass">)  [unwired: 7 in]
            n133 = Bundle("Output Array"=w363, dbl[] [0.1, 0.1, 0.1, 0.1]) -> (w361:cluster{"Output Array":string[], dbl[]})  [unwired: 1 in]
            n134 = Multiply(x=1000.0, y=w377) -> (x*y=w360:dbl[])
            n135 = Bundle By Name(cluster=T6 {"PT +Channels"=["AIN0", "AIN2", "AIN4", "AIN6"], "PT -Channels"=[1, 3, 5, 7], "PT Multipliers"=[], "PT Offsets"=[]}, "PT Multipliers"=w360, "PT Offsets"=w376) -> (w375:T6)
            n136 = call "Send Message.vim"("error in (no error)"=w393, "Contents"=w361, "Label or Message"="eWriteNames", "Address"=w368) -> ("error out"=w369:errorcluster, "Address out"=w367:refnum<class "Actor type2.lvclass">)  [unwired: 6 in]
            n137 = call "Send Message.vim"("error in (no error)"=w369, "Contents"=w375, "Label or Message"="Setup Diff PTs", "Address"=w367) -> ("error out"=w385:errorcluster)  [unwired: 6 in, 1 out]
            n138 = Get Date/Time In Seconds() -> (seconds since 1Jan1904=w388:timestamp)
            n139 = call <vilib>:"Set Period.vi"("error in (no error)"=w385, "Period (ms)"=w372, "Metronome in"=w373) -> ("error out"=w374:errorcluster)  [unwired: 7 in, 1 out]
            n140 = Divide(x=w372, y=1000) -> (x/y=w370:dbl)
            n141 = Bundle By Name(cluster=w392, "LabJack.t0"=w388, "LabJack.PT Names"=w379, "LabJack.dt"=w370) -> (w389:T3)
          }
          frame "LabJack:UpdateReg" {
            n142 = Variant To Data(error in=w408, type=0.0, Variant=w406) -> (data=w397:dbl, error out=w407:errorcluster)
            n143 = Unbundle By Name(w403) -> ("LabJack.Actor"=w402:refnum<class "Actor type2.lvclass">, "LabJack.TDAC#"=w400:string)
            n144 = Divide(x=w397, y=45.0) -> (x/y=w395:dbl)
            n145 = Bundle("TDAC#"=w400, w395) -> (w399:cluster{"TDAC#":string, dbl})  [unwired: 1 in]
            n146 = call "Send Message.vim"("error in (no error)"=w407, "Contents"=w399, "Label or Message"="eWriteName", "Address"=w402) -> ("error out"=w404:errorcluster)  [unwired: 6 in, 1 out]
            n147 = Bundle By Name(cluster=w403, "LabJack.Target PSI"=w397) -> (w398:T3)
          }
          frame "LabJack:Data" {
            n148 = Unbundle By Name(w422) -> ("LabJack.PT Data"=w427:dbl[][], "DataLogger.Actor"=w424:refnum<class "Actor type2.lvclass">, "DataLogger.Data Packet"=w421:T7, "LabJack.t0"=w412:timestamp, "LabJack.dt"=w411:dbl, "LabJack.PT Names"=w414:string[], "LabJack.Target PSI"=w413:dbl)
            n149 = Variant To Data(error in=w430, type=dbl[] [], Variant=w429) -> (data=w415:dbl[], error out=w428:errorcluster)
            n150 = Build Array (concatenate)(w413, w415) -> (w409:dbl[])
            n151 = Build Array (concatenate)(w427, w409) -> (w417:dbl[][])
            n152 = Bundle By Name(cluster=w421, "Group Name"="PT Data", "Channel Names"=w414, "Data"=w409) -> (w420:T7)
            n153 = Transpose 2D Array(2D array=w417) -> (transposed array=w416:dbl[][])
            n154 = for {
              tunnel: w416 -> [w431] mode=indexing
              tunnel: w412 -> [w434]
              tunnel: w411 -> [w433]
              tunnel: [w432] -> w410 mode=indexing
              tunnel: [w431] -> _
              n155 = Bundle By Name("Y"=w431, "t0"=w434, "dt"=w433) -> (w432:waveform(dbl))  [unwired: 1 in]
            }
            n156 = call "Send Message.vim"("error in (no error)"=w428, "Contents"=w420, "Label or Message"="Write Data", "Address"=w424) -> ("error out"=w425:errorcluster)  [unwired: 6 in, 1 out]
            n157 = Bundle By Name(cluster=w422, "LabJack.PT Data"=w417, "App Control.WFM Data"=w410, "App Control.PT Data"=w409) -> (w426:T3)
          }
          frame "------Test Actions------" {
          }
          frame "Test Status" {
            n158 = Unbundle By Name(w441) -> ("Test Status.Test Status"=w437:string)
            n159 = case shown="\"Idle\", Default" w437 {
              tunnel: w441 -> [w443]
              tunnel: [w443] -> w440
              tunnel: w439 -> [w442]
              tunnel: [w442] -> w438
              frame "Idle", Default {
              }
            }
          }
          frame "------App Control------" {
          }
          frame "Update FP" {
            n160 = Unbundle By Name(w448) -> ("App Control.PT Data"=w447:dbl[], "App Control.WFM Data"=w446:waveform(dbl)[])
            n161 = call "PressuresFP.vi"("Array"=w446, "Pressures"=w447) -> ()  [unwired: 10 in]
          }
          frame "Front Panel Config" {
            n162 = Unbundle By Name(w459) -> ("App Control.This VI"=w453:refnum<vi>, "App Control.Front Panel Config refnum"=w452:T2)
            n163 = Variant To Data(error in=w461, type=TRUE, Variant=w457) -> (data=w455:bool, error out=w458:errorcluster)
            n164 = Build Array(refnum<vi> refnum ("reference out")) -> (w463:refnum<vi>[])
            n165 = for {
              shift-right: [w467] -> w464
              shift-left: w458 -> [w470]
              tunnel: w463 -> [w468] mode=indexing
              tunnel: [w465] -> w462 mode=indexing
              n166 = property on="Property Node" class="Ctl"(reference=w468, error in=w470) -> (reference out=w466:refnum<vi>, error out=w469:errorcluster, "Label.Text"=w465:string)
              n167 = Close Reference(reference=w466, error in (no error)=w469) -> (error out=w467:errorcluster)
            }
            n168 = case shown="False" w455 {
              tunnel: [w474 w481] -> w460
              tunnel: w464 -> [w475 w480]
              tunnel: w452 -> [w472 w477]
              tunnel: w453 -> [w471 w476]
              tunnel: [w473 w479] -> w450
              tunnel: w462 -> [_ w478]
              frame False {
                n169 = call "Write Panel Controls to INI.vi"("error in (no error)"=w475, "VI ref"=w471, "refnum"=w472) -> ("error out"=w474:errorcluster, "refnum out"=w473:T2)  [unwired: 7 in]
              }
              frame True {
                n170 = call "Read Panel Controls.vi"("error in (no error)"=w480, "Skip Controls"=w478, "VI ref"=w476, "refnum"=w477) -> ("error out"=w481:errorcluster, "refnum out"=w479:T2)  [unwired: 6 in]
              }
            }
            n171 = Bundle By Name(cluster=w459, "App Control.Front Panel Config refnum"=w450) -> (w451:T3)
          }
          frame "EmailNotification" {
            n172 = Unbundle By Name(w489) -> ("EmailNotifier.Actor"=w488:refnum<class "Actor type2.lvclass">)
            n173 = call "Send Message.vim"("error in (no error)"=w491, "Contents"="philip.thiessen@orbitfab.com", "Label or Message"="Set Recipeints", "Address"=w488) -> ("error out"=w490:errorcluster, "Address out"=w484:refnum<class "Actor type2.lvclass">)  [unwired: 6 in]
            n174 = call "Send Message.vim"("error in (no error)"=w490, "Contents"=cluster{"Subject":string, "Message":string} {"Subject"="Test Notification", "Message"="Test Notification"}, "Label or Message"="Send Email", "Address"=w484) -> ("error out"=w485:errorcluster)  [unwired: 6 in, 1 out]
          }
        }
      }
      frame Error {
        n175 = Bundle By Name(cluster=w495, "Event"="Cleanup") -> (w499:cluster{"Event":string, "Data":variant})
        n176 = Unbundle By Name(w501) -> ("TopLevelMessenger"=w494:refnum<class "EventMessenger.lvclass">)
        n177 = Enqueue Element(queue=w492, element=w499) -> (error out=w500:errorcluster)  [unwired: 2 in, 2 out]
        n178 = call "Send Message.vim"("error in (no error)"=w500, "Contents"=w496, "Label or Message"="Consumer Error", "Address"=w494) -> ("error out"=w493:errorcluster)  [unwired: 6 in, 1 out]
      }
    }
  }
  n179 = Merge Errors(w13, w14) -> (w12:errorcluster)
  n180 = Release Queue(queue=w11, error in (no error)=w12) -> (error out=w10:errorcluster)  [unwired: 1 in, 2 out]
  n181 = call <vilib>:"Simple Error Handler.vi"("error in (no error)"=w10) -> ()  [unwired: 4 in, 5 out]
